vi "查找替换数组元素(1D I8).vi"(7 "开始索引（0）":i32, 8 "error in (no error)":errorcluster caption="错误输入（无错误）", 9 "替换值":i8, 10 "查找元素":i8, 11 "输入数组":i8[](array[numeric])) -> (0 "error out":errorcluster caption="错误输出", 2 "替换索引":i32[](array[numeric]), 3 "输出数组":i8[](array[numeric]))   [LabVIEW 2012]
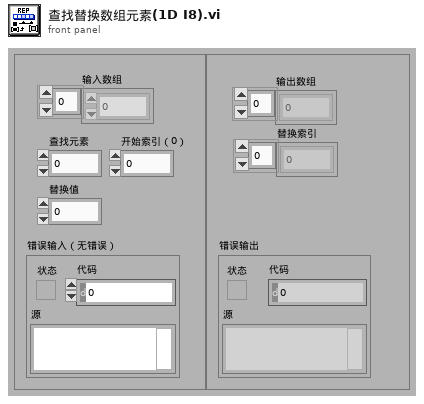
[diagram p1: front panel]
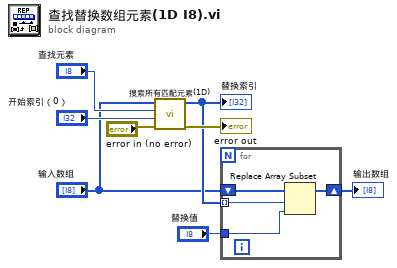
[diagram p0: block diagram]
diagram:
  n1 = call-poly "搜索所有匹配元素(1D).vi"("error in (no error)"="error in (no error)", "开始索引（0）"="开始索引（0）", "元素"="查找元素", "数组"="输入数组") -> ("error out"=→"error out":errorcluster, "匹配元素索引"=w4:i32[])  [unwired: 5 in, 1 out]
  "替换索引" <- w4
  n2 = for {
    tunnel: w4 -> [w10] mode=indexing
    shift-right: [w11] -> w2
    shift-left: "输入数组" -> [w12]
    tunnel: "替换值" -> [w9]
    n3 = Replace Array Subset(array=w12, new element=w9, index=w10) -> (w11:i8[])
  }
  "输出数组" <- w2
